vi "Page_Info_Write.vi"(6 "ctlReferences":T1, 8 "error in (no error)":errorcluster, 10 "Target filename":string, 11 "AB_WebService in":refnum<class "AB_WebService.lvclass">) -> (0 "error out":errorcluster, 3 "AB_WebService out":refnum<class "AB_WebService.lvclass">)   [LabVIEW 2020, in "AB_WebService.lvclass"]
uses:
  <vilib>/AppBuilder/AB_Classes/WebService/AB_WebService.lvclass
  <resource>/Framework/Providers/Builds/AppBuilder/AB_UI_Page_Info_References.ctl
  <vilib>/AppBuilder/AB_Classes/TargetFile/AB_Targetfile.lvclass
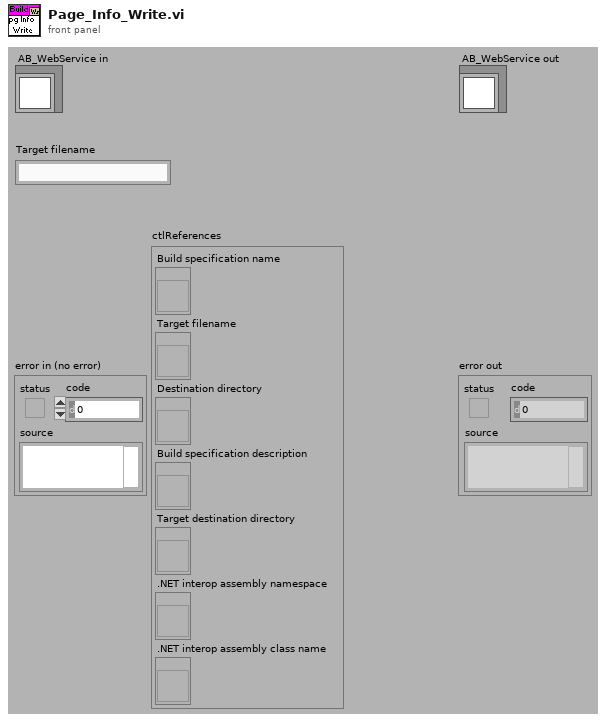
[diagram p1: front panel]
types:
  T1 = typedef "AB_UI_Page_Info_References.ctl" = cluster{"Build specification name":refnum<vi>, "Target filename":refnum<vi>, "Destination directory":refnum<vi>, "Build specification description":refnum<vi>, "Target destination directory":refnum<vi>, ".NET interop assembly namespace":refnum<vi>, ".NET interop assembly class name":refnum<vi>}
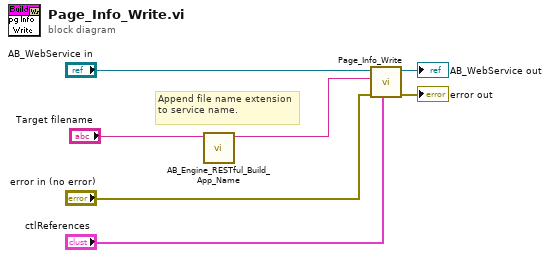
[diagram p0: block diagram]
diagram:
  # "Append file name extension to service name."
  n1 = call <vilib>:"AB_Engine_RESTful_Build_App_Name.vi"("service name"="Target filename") -> ("app name"=w1:string)  [unwired: 10 in]
  n2 = call-parent "Page_Info_Write.vi"("ctlReferences"="ctlReferences", "error in (no error)"="error in (no error)", "Target filename"=w1, "AB_Targetfile in"="AB_WebService in") -> ("error out"=→"error out":errorcluster, "AB_Targetfile out"=→"AB_WebService out":refnum<class "AB_WebService.lvclass">)  [unwired: 6 in]
